vi "Preset Expt Device Comparison.vi"(8 "Input Type":enum16{"Preset Queue", "Preset Only"}(ring), 9 "Preset Name":string, 10 "Preset Array":string[][](array[string]), 11 "Expt name":string) -> (1 "Devices Not in Experiment":string[](array[string]), 3 "Devices accounted for?":bool)   [LabVIEW 2020]
uses:
  Shared/MySQL/Preset Query Enum.ctl
  5c59b56e-ab11-48a6-a012-8629b329c53a.vi
  101616bc-c781-4ec3-be02-7ffc3d1c27c7.vi
panel:
  out "String":string
  out "device list":string[](array[string])
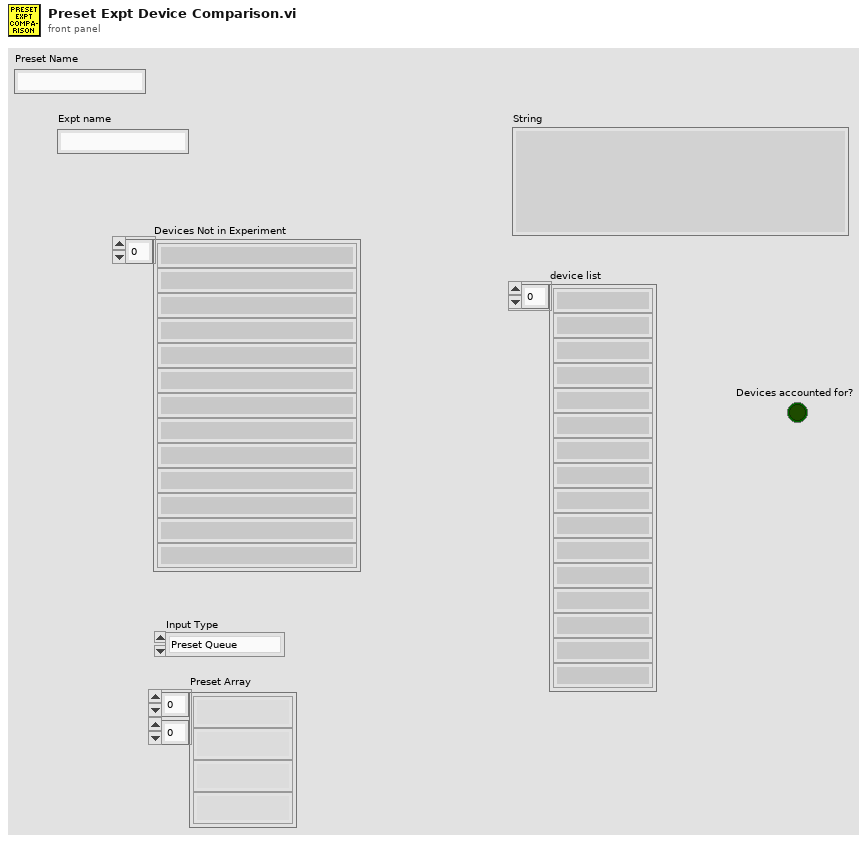
[diagram p1: front panel]
types:
  T1 = typedef "Preset Query Enum.ctl" = enum16{"Get Locations", "Get all IPs and MACs", "Get classes", "Get expt variables to set at scanstart for particular device", "Get expt devices and variables with start values", "Get expt devices and variables (with data to get)", "Get expt devices with data to get", "Get Expt devices and GUIs", "Get all devices basic properties", "Get Virtual Devices Core Info", "Get Expt names", "Get experiment basic properties", "Get experiment alarm variables", "Get MC Ports", "Get device network comm port", "Get devicetype lvclass path", "Get basic device properties", "Get Init Order", "Get all setable variables of a device", "Get device variable aliases", "Get force values of all settable variables", "Get all variables of a devicetype", "Get all variables of a device", "Get plotter details", "Get Saved Scans", "Get Scan Info", "GetGeneralGUIs", "Get expt for plotter", "Get plotter IDs from expt", "Get all devices", "Get all Virtual Devices", "Get all aliases", "Get variable and device info for Virtual Device", "GetItemLocatorIP", "Get IPs for GUIs", "Get DeviceType from Device", "GetLocalPortRange", "GetDevicePresetVariables", "Get Device Configuration", "GetAllPresetNames", "GetAllConfigurationNames", "GetPresetDeviceNames", "GetDeviceAliases", "GetDevicesOfClass"}
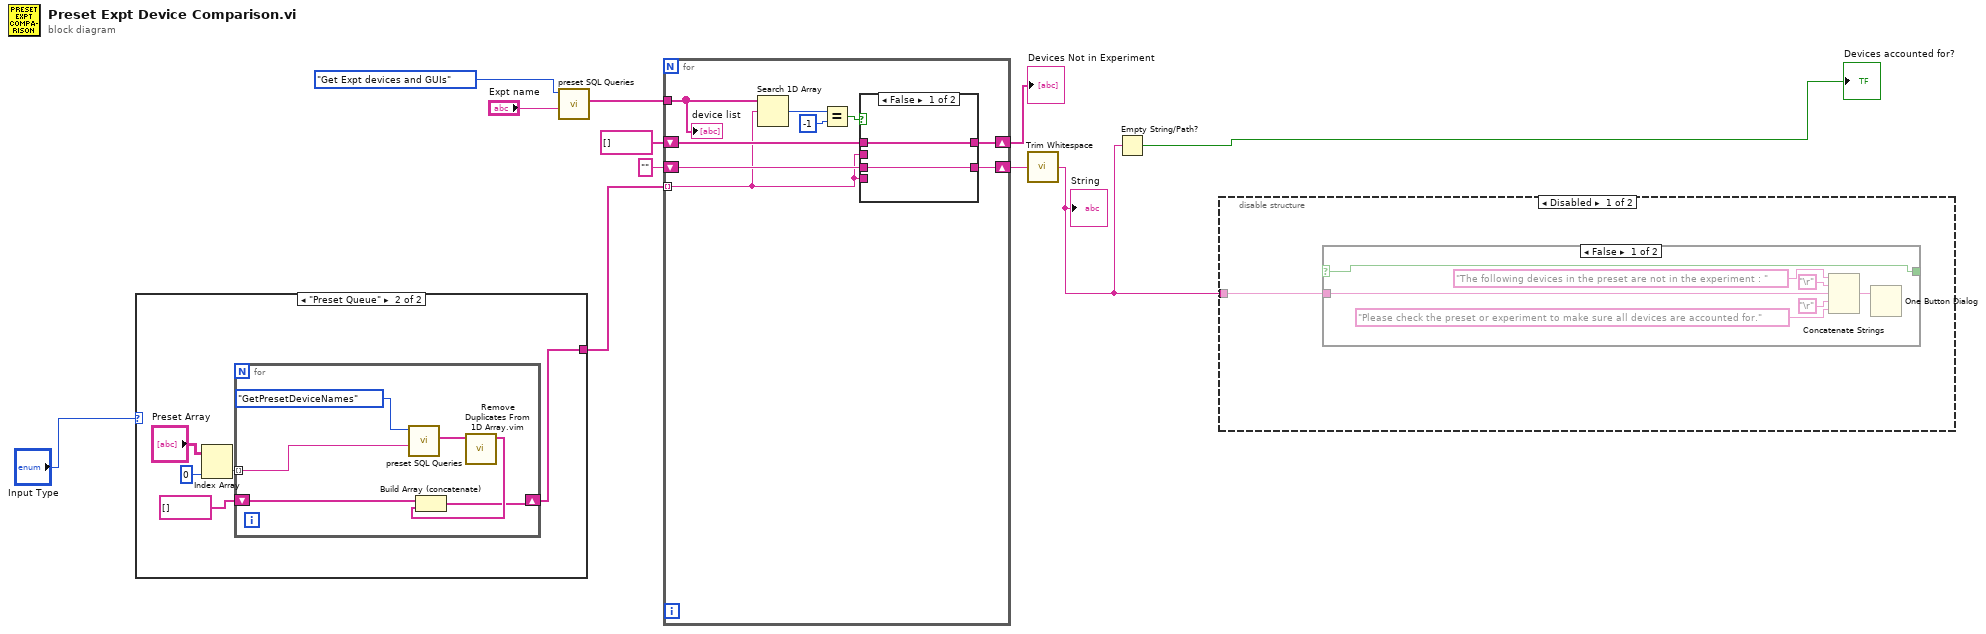
[diagram p0: block diagram]
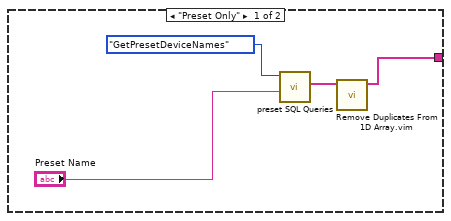
[diagram p4: hidden frame]
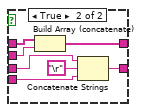
[diagram p5: hidden frame]
diagram:
  n1 = case shown="\"Preset Queue\"" "Input Type" {
    tunnel: [w15 w16] -> w8
    frame "Preset Only" {
      n2 = call "preset SQL Queries.vi"("Expt name / MCIP/ Variable/Preset Name"="Preset Name", "Preset Query"=Preset_Query_Enum."GetPresetDeviceNames") -> ("1st column 1st data"=w13:string[])  [unwired: 7 in, 2 out]
      n3 = call "Remove Duplicates From 1D Array.vim"("array"=w13) -> ("array with duplicates removed"=w15:string[])  [unwired: 10 in]
    }
    frame "Preset Queue" {
      n4 = Index Array(array="Preset Array", index (col)=0 ("disabled index (col)")) -> (element=w18:string[])  [unwired: 1 in]
      n5 = for {
        tunnel: w18 -> [w24] mode=indexing
        shift-right: [w21] -> w16
        shift-left: string[] [] -> [w23]
        n6 = call "preset SQL Queries.vi"("Expt name / MCIP/ Variable/Preset Name"=w24, "Preset Query"=Preset_Query_Enum."GetPresetDeviceNames") -> ("1st column 1st data"=w26:string[])  [unwired: 7 in, 2 out]
        n7 = call "Remove Duplicates From 1D Array.vim"("array"=w26) -> ("array with duplicates removed"=w22:string[])  [unwired: 10 in]
        n8 = Build Array (concatenate)(w23, w22) -> (w21:string[])
      }
    }
  }
  n9 = call "preset SQL Queries.vi"("Expt name / MCIP/ Variable/Preset Name"="Expt name", "Preset Query"=Preset_Query_Enum."Get Expt devices and GUIs") -> ("1st column 1st data"=w9:string[])  [unwired: 7 in, 2 out]
  n10 = for {
    tunnel: w9 -> [w35]
    tunnel: w8 -> [w28] mode=indexing
    shift-right: [w30] -> w6
    shift-left: "" -> [w31]
    shift-right: [w27] -> w3
    shift-left: string[] [] -> [w29]
    n11 = Search 1D Array(1D array=w35, element=w28) -> (index of element=w34:i32)  [unwired: 1 in]
    n12 = Equal?(x=w34, y=-1) -> (x = y?=w32:bool)
    n13 = case shown="False" w32 {
      tunnel: w31 -> [w37 w44]
      tunnel: [w37 w43] -> w30
      tunnel: w28 -> [_ w42]
      tunnel: w29 -> [w36 w40]
      tunnel: w28 -> [_ w39]
      tunnel: [w36 w38] -> w27
      frame False {
      }
      frame True {
        n14 = Build Array (concatenate)(w40, w39) -> (w38:string[])
        n15 = Concatenate Strings(w44, "\r", w42) -> (w43:string)
      }
    }
    "device list" <- w35
  }
  "Devices Not in Experiment" <- w3
  n16 = call <vilib>:"Trim Whitespace.vi"("string"=w6) -> ("trimmed string"=w5:string)  [unwired: 1 in]
  "String" <- w5
  n17 = Empty String/Path?(string/path=w5) -> (empty?=→"Devices accounted for?":bool)
  n18 = disable-structure shown="Disabled" {
    disable-tunnel: w5 -> [w45 _]
    frame Disabled {
      n19 = case shown="False" {
        selector: _ -> [w46 w53]
        tunnel: [w46 w53] -> _
        tunnel: w45 -> [w50 _]
        frame False {
          n20 = Concatenate Strings("The following devices in the preset are not in the experiment : ", "\r", w50, "\r", "Please check the preset or experiment to make sure all devices are accounted for." ("string")) -> (w47:string)
          n21 = One Button Dialog(message=w47) -> ()  [unwired: 1 in, 1 out]
        }
        frame True {
        }
      }
    }
    frame Enabled {
    }
  }
